vi "GetEvtSignal.vi"(8 "error in (no error)":errorcluster, 11 "C37EventPlugin in":refnum<class "UserEvtPlugins.lvclass">) -> (0 "error out":errorcluster, 3 "C37EventPlugin out":refnum<class "UserEvtPlugins.lvclass">)   [LabVIEW 2017, in "EventPlugins.lvlib" / "UserEvtPlugins.lvclass"]
uses:
  UserEvtPlugins.lvclass
  C:/dev/Work/PARTF/Modules/EventPlugins/EventPluginBaseClass/EventPluginBaseClass.lvclass
  C:/Program Files (x86)/National Instruments/LabVIEW 2017/user.lib/NIST/BaseClasses/BasePlugin_class/BasePlugin.lvclass
  <userlib>/NIST/BaseClasses/BasePlugin_class/BasePlugin.lvclass/BasePlugin.ctl
  <userlib>/NIST/BaseClasses/BasePlugin_class/Accessors/Read PluginIniFilePath.vi
  EventPluginBaseClass/Accessors/Read EvtConfig.vi
  EventPluginBaseClass/Accessors/Read TimeArray.vi
  EventPluginBaseClass/Accessors/Read EvtParams.vi
  <vilib>/Utility/config.llb/Read Key (String).vi
  <vilib>/Utility/config.llb/NI_LVConfig.lvlib
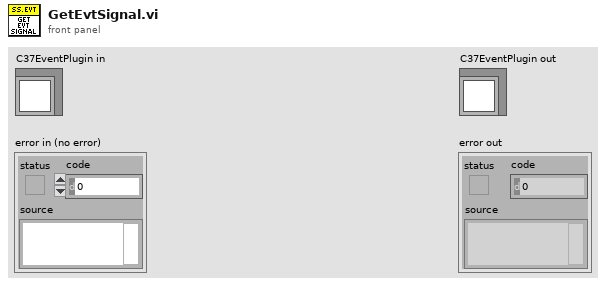
[diagram p1: front panel]
types:
  T1 = typedef "EventPlugins.lvlib/EventPluginBaseClass.lvclass/clEvtConfig.ctl" = cluster{"T0(UTC)":dbl, "F0":dbl, "Fs":i32, "FSamp":u32, "bPosSeq":bool}
  T2 = typedef "NI_LVConfig.lvlib/Config Data RefNum.ctl" = refnum<k1>
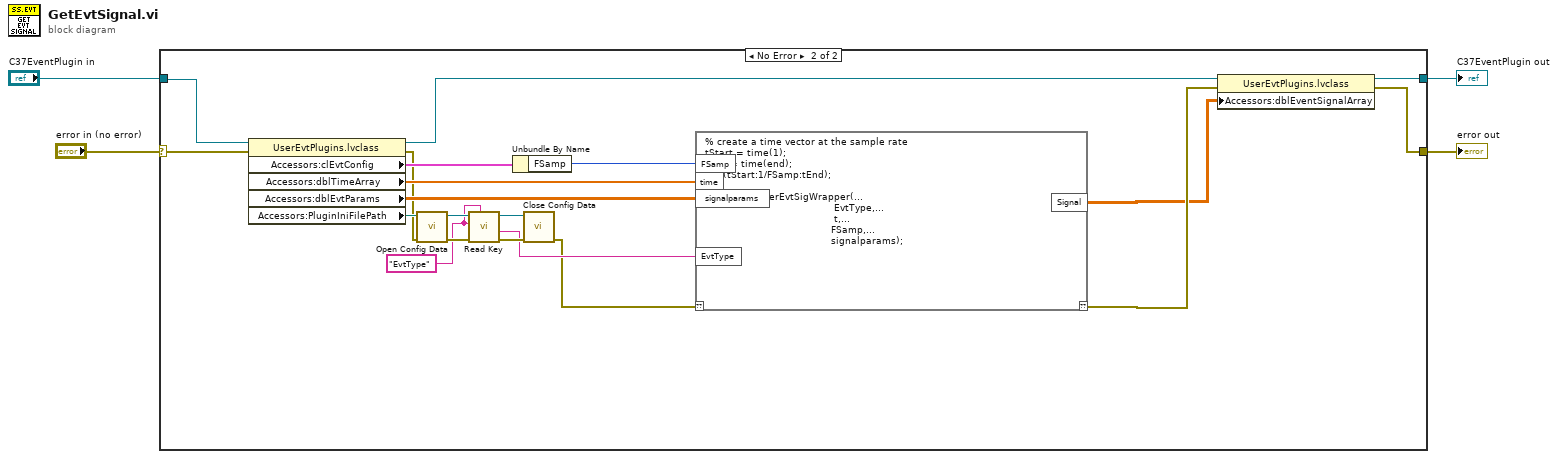
[diagram p0: block diagram]
diagram:
  n1 = case shown="No Error" "error in (no error)" {
    selector: "error in (no error)" -> [w6 w23]
    tunnel: [w5 w26] -> w4
    tunnel: "C37EventPlugin in" -> [w5 w24]
    tunnel: [w6 w25] -> w3
    frame Error {
    }
    frame No Error {
      w11 = "EvtType" ("section")
      n2 = property class="UserEvtPlugins.lvclass"(reference=w24, error in=w23) -> (reference out=w20:refnum<class "UserEvtPlugins.lvclass">, error out=w14:errorcluster, "Accessors:clEvtConfig"=w22:T1, "Accessors:dblTimeArray"=w18:dbl[], "Accessors:dblEvtParams"=w17:dbl[][], "Accessors:PluginIniFilePath"=w15:path)
      n3 = call <vilib>:"Open Config Data.vi"("error in (no error)"=w14, "configuration file path"=w15) -> ("error out"=w13:errorcluster, "refnum"=w12:T2)  [unwired: 7 in, 1 out]
      n4 = call-poly <vilib>:"Read Key.vi"("section"=w11, "error in (no error)"=w13, "key"=w11, "refnum"=w12) -> ("error out"=w10:errorcluster, "value"=w8:string, "refnum out"=w9:T2)  [unwired: 4 in, 1 out]
      n5 = Unbundle By Name(w22) -> ("FSamp"=w21:u32)
      n6 = call <vilib>:"Close Config Data.vi"("error in (no error)"=w10, "refnum"=w9) -> ("error out"=w7:errorcluster)  [unwired: 8 in, 1 out]
      n7 = script code="% create a time vector at the sample rate\ntStart = time(1);\ntEnd = time(end);\nt = (tStart:1/FSamp:tEnd);\n\n[Signal] = UserEvtSigWrapper(...\n                                           EvtType,...\n                                           t,...\n                                          FSamp,...\n                                          signalparams);"("??"=w7, "FSamp"=w21, "time"=w18, "signalparams"=w17, "EvtType"=w8) -> ("??"=w19:errorcluster, "Signal"=w16:dbl[][])
      n8 = property class="UserEvtPlugins.lvclass"(reference=w20, error in=w19, "Accessors:dblEventSignalArray"=w16) -> (reference out=w26:refnum<class "UserEvtPlugins.lvclass">, error out=w25:errorcluster)
    }
  }
  "error out" <- w3
  "C37EventPlugin out" <- w4
